vi "uTTA_Calibration_DiffAmp.vi"(6 "AR488_in":refnum<visa-resource-name>, 7 "CommandQueue":refnum<queue>, 8 "error in":errorcluster, 9 "FunctionGen_In":refnum<visa-resource-name>, 10 "DataQueue":refnum<queue>, 11 "TDMS_FileIn":refnum<k34>) -> (0 "error out":errorcluster, 1 "FunctionGen_Out":refnum<visa-resource-name>, 2 "aborted":bool, 3 "TDMS_FileOut":refnum<k34>, 4 "AR488_out":refnum<visa-resource-name>)   [LabVIEW 2021]
uses:
  <vilib>/Utility/miscctls.llb/LVPointTypeDef.ctl
  <vilib>/Analysis/6fits.llb/Curve Fitting Criteria.ctl
  <vilib>/Analysis/NI_AALPro.lvlib
panel:
  in  "START":bool
  out "ADC_Values":dbl[](array[numeric]) format="%#.2g"
  out "ADC_Variance":dbl[](array[numeric]) format="%#.2g"
  out "ADC offset":dbl format="%#_6pV"
  out "ADC lin. res":dbl caption="Residue" format="%.3p"
  out "ADC slope":dbl format="%#_4pV/Digit"
  out "Ref. Voltage":dbl format="%#_6pV"
  out "ADC Cal.":cluster{"mean":dbl, "mean":dbl}(graph)
  out "PGA setting":u32
  out "Calibration of Channel":u32
  in  "DAC Increments":dbl=0.05 caption="DAC Voltage Increment" min=0.001 max=1.0 format="%.3p V/Step"
  in  "Cal Adapter":bool=TRUE
  out "Status":string="Exit"
  in  "abort":bool
  # "1. Connect the function generator with a 50Ohm Terminator and a BNC Y-Adaptor to the input of the uTTA.\n2. Connect a ground lead to the outer Conductor of the BNC line to provide propper grounding\n3. Start the calibration"
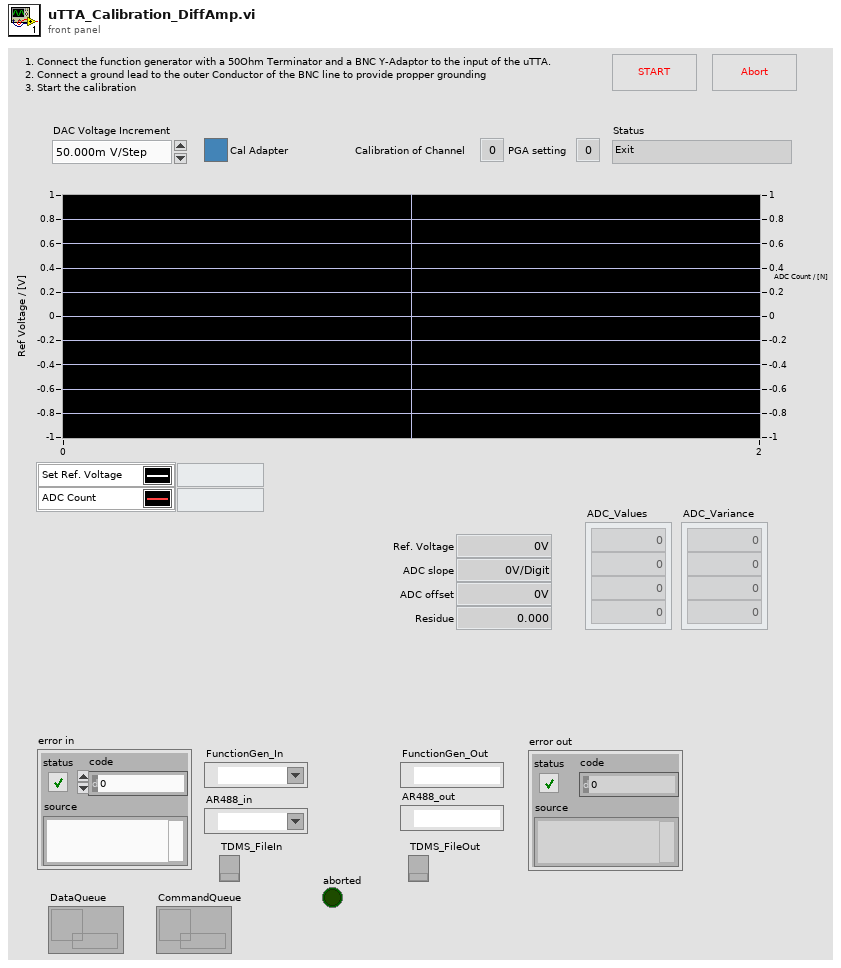
[diagram p1: front panel]
types:
  T1 = typedef "LVPointTypeDef.ctl" = cluster{"Horizontal":i16, "Vertical":i16}
  T2 = typedef "NI_AALPro.lvlib/Curve Fitting Criteria.ctl" = u16
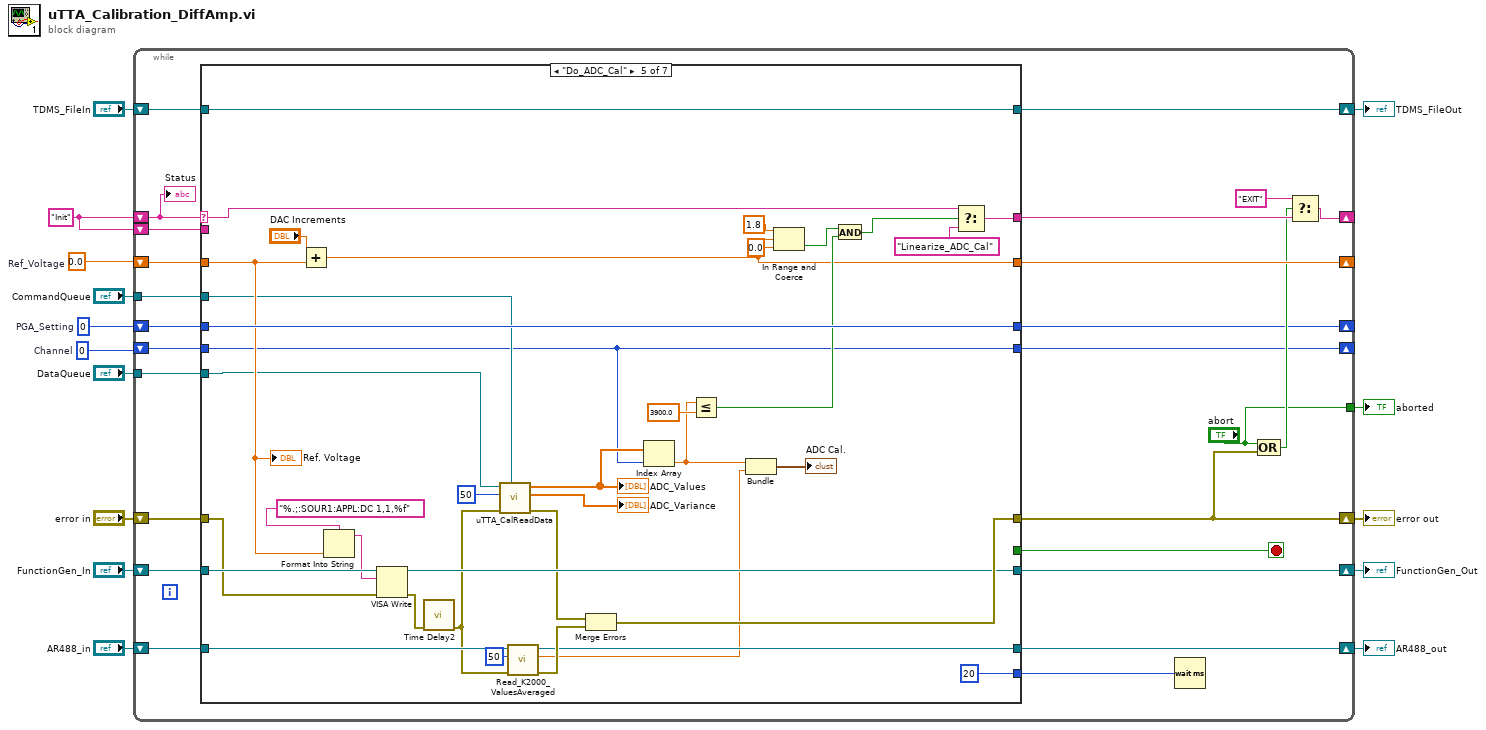
[diagram p0: block diagram]
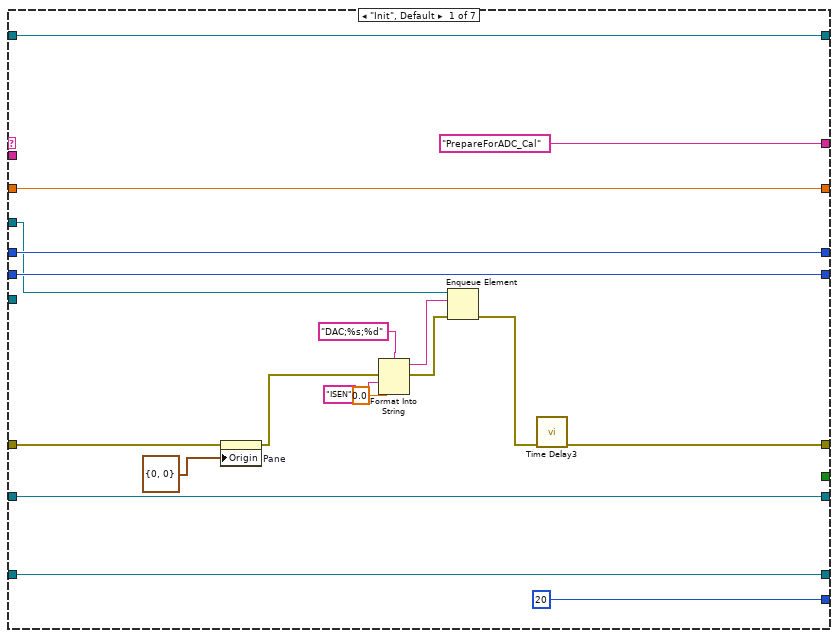
[diagram p2: hidden frame]
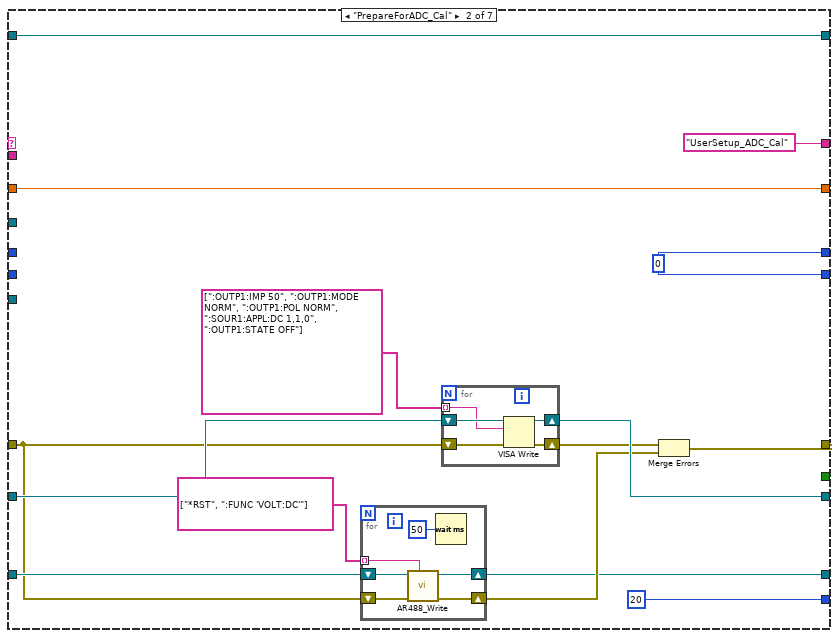
[diagram p3: hidden frame]
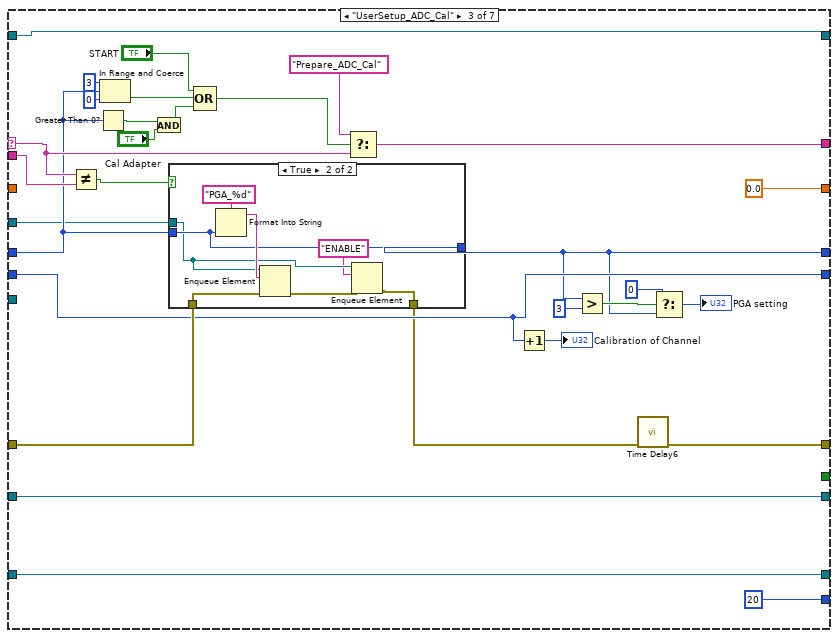
[diagram p4: hidden frame]
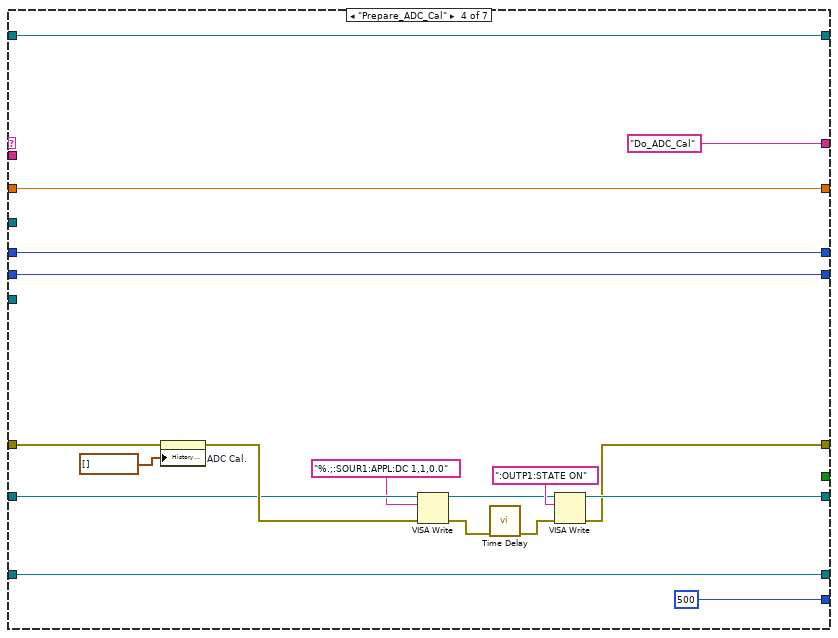
[diagram p6: hidden frame]
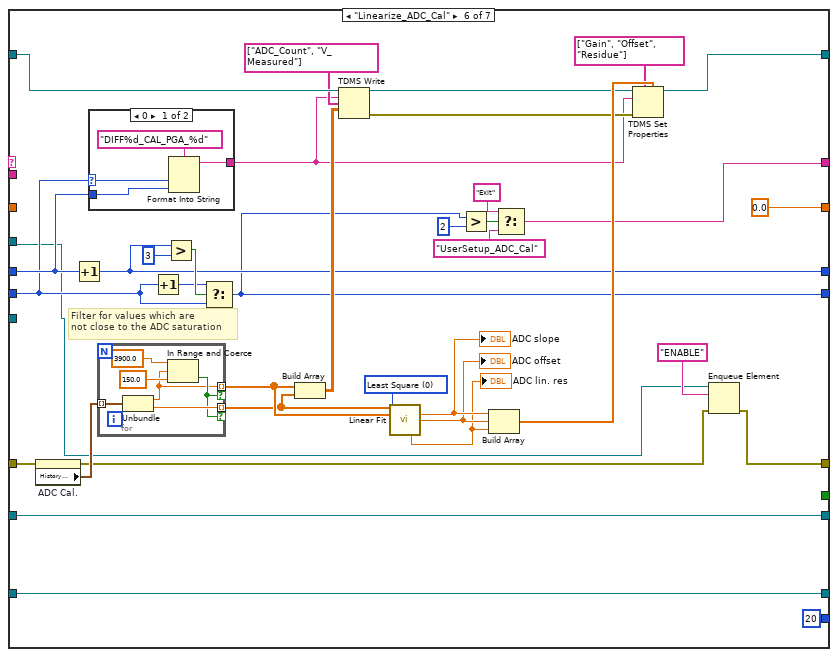
[diagram p7: hidden frame]
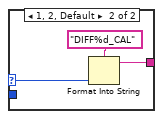
[diagram p8: hidden frame]
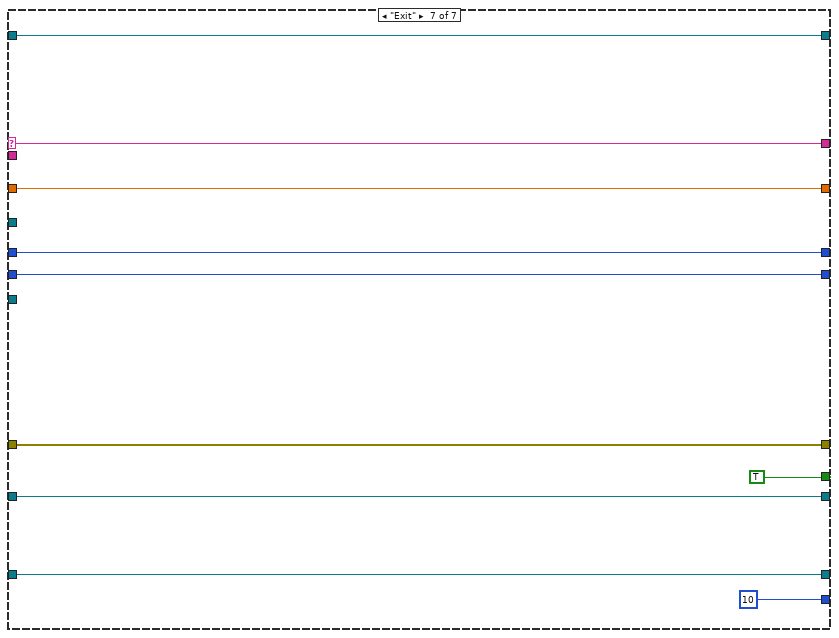
[diagram p9: hidden frame]
diagram:
  w11 = 0  # Channel
  w12 = 0  # PGA_Setting
  w14 = 0.0  # Ref_Voltage
  w13 = "Init"
  n1 = while {
    shift-right: [w27] -> _
    shift-left: w13 -> [w38]
    shift-right: [w25] -> w15
    shift-left: "error in" -> [w40]
    shift-right: [w36] -> w3
    shift-left: "FunctionGen_In" -> [w37]
    shift-right: [w35] -> w2
    shift-left: "AR488_in" -> [w34]
    shift-left: w13 -> [w33]
    tunnel: "CommandQueue" -> [w32]
    tunnel: "DataQueue" -> [w31]
    shift-right: [w29] -> _
    shift-left: w14 -> [w30]
    shift-right: [w22] -> w7
    shift-left: "TDMS_FileIn" -> [w21]
    shift-right: [w19] -> _
    shift-left: w12 -> [w20]
    shift-right: [w17] -> _
    shift-left: w11 -> [w18]
    tunnel: ["abort"] -> w1
    stop <- w23 stop-if-true
    n2 = case shown="\"Do_ADC_Cal\"" w38 {
      selector: w38 -> [_ _ w100 _ w175 _ w240]
      tunnel: [_ _ _ _ _ _ TRUE] -> w23
      tunnel: w40 -> [w56 w62 w108 w139 w165 w211 w234]
      tunnel: ["PrepareForADC_Cal" ("t") "UserSetup_ADC_Cal" ("t") w115 "Do_ADC_Cal" ("t") w174 w187 w240] -> w28
      tunnel: [w41 w71 w96 w135 w173 w183 w234] -> w25
      tunnel: [u32 20 u32 20 u32 20 u32 500 u32 20 u32 20 u32 10] -> w39
      tunnel: w37 -> [w55 w63 w114 w130 w166 w215 w233]
      tunnel: [w55 w73 w114 w136 w164 w215 w233] -> w36
      tunnel: [w54 w66 w113 w142 w169 w213 w232] -> w35
      tunnel: w34 -> [w54 w65 w113 w142 w171 w213 w232]
      tunnel: w33 -> [_ _ w99 _ _ _ _]
      tunnel: w32 -> [w43 _ w87 _ w145 w181 _]
      tunnel: w31 -> [_ _ _ _ w152 _ _]
      tunnel: w30 -> [w53 w70 _ w140 w154 _ w237]
      tunnel: [w53 w70 0.0 w140 w153 0.0 w237] -> w29
      tunnel: [w52 w64 w109 w138 w167 w209 w236] -> w22
      tunnel: w21 -> [w52 w64 w109 w138 w167 w210 w236]
      tunnel: w20 -> [w50 _ w94 w134 w159 w192 w231]
      tunnel: [w50 w60 w97 w134 w159 w199 w231] -> w19
      tunnel: w18 -> [w51 _ w104 w132 w144 w190 w235]
      tunnel: [w51 w60 w104 w132 w144 w188 w235] -> w17
      frame "Init", Default {
        n3 = property on="Pane" class="Pane"(error in=w56, "Origin"=T1 {"Horizontal"=0, "Vertical"=0}) -> (error out=w45:errorcluster)  [unwired: 1 in, 1 out]
        n4 = Format Into String(format string="DAC;%s;%d" ("element"), error in=w45, "ISEN" ("input 1"), 0.0 ("input 2")) -> (resulting string=w49:string, error out=w48:errorcluster)  [unwired: 1 in]
        n5 = Enqueue Element(queue=w43, element=w49, error in (no error)=w48) -> (error out=w42:errorcluster)  [unwired: 1 in, 2 out]
        n6 = call "Time Delay3"("error in (no error)"=w42) -> ("error out"=w41:errorcluster)  [unwired: 10 in]
      }
      frame "PrepareForADC_Cal" {
        w60 = 0 ("Channel")
        n7 = for {
          tunnel: string[] ["*RST", ":FUNC 'VOLT:DC'"] -> [w79] mode=indexing
          shift-right: [w77] -> w66
          shift-left: w65 -> [w80]
          shift-right: [w76] -> w67
          shift-left: w62 -> [w78]
          n8 = call "AR488_Write.vi"("write"=w79, "error in (no error)"=w78, "VISA Refnum in"=w80) -> ("error out"=w76:errorcluster, "VISA Refnum out"=w77:refnum<visa-resource-name>)  [unwired: 7 in]
          n9 = Wait (ms)(milliseconds to wait=u32 50) -> ()  [unwired: 1 out]
        }
        n10 = for {
          shift-right: [w84] -> w73
          shift-left: w63 -> [w85]
          tunnel: string[] [":OUTP1:IMP 50", ":OUTP1:MODE NORM", ":OUTP1:POL NORM", ":SOUR1:APPL:DC 1,1,0", ":OUTP1:STATE OFF"] ("Array 2") -> [w83] mode=indexing
          shift-right: [w81] -> w72
          shift-left: w62 -> [w82]
          n11 = VISA Write(VISA resource name=w85, write buffer=w83, error in (no error)=w82) -> (VISA resource name out=w84:refnum<visa-resource-name>, error out=w81:errorcluster)  [unwired: 1 out]
        }
        n12 = Merge Errors(w72, w67) -> (w71:errorcluster)
      }
      frame "UserSetup_ADC_Cal" {
        n13 = Not Equal?(x=w100, y=w99) -> (x != y?=w98:bool)
        n14 = Greater Than 0?(x=w94) -> (x > 0?=w92:bool)
        n15 = In Range and Coerce(upper limit=u32 3, x=w94, lower limit=u32 0) -> (In Range?=w101:bool)  [unwired: 1 out]
        n16 = And(x=w92, y="Cal Adapter") -> (x .and. y?=w91:bool)
        n17 = case shown="True" w98 {
          tunnel: w108 -> [w116 w125]
          tunnel: w87 -> [_ w121]
          tunnel: w94 -> [w117 w122]
          tunnel: [w117 w122] -> w97
          tunnel: [w116 w118] -> w86
          frame False {
          }
          frame True {
            n18 = Format Into String(format string="PGA_%d" ("element"), w122) -> (resulting string=w123:string)  [unwired: 2 in, 1 out]
            n19 = Enqueue Element(queue=w121, element=w123, error in (no error)=w125) -> (error out=w119:errorcluster)  [unwired: 1 in, 2 out]
            n20 = Enqueue Element(queue=w121, element="ENABLE", error in (no error)=w119) -> (error out=w118:errorcluster)  [unwired: 1 in, 2 out]
          }
        }
        n21 = Compound Arithmetic op=OR("START", w101, w91) -> (w103:bool)
        n22 = Select(t="Prepare_ADC_Cal", s=w103, f=w100) -> (s? t:f=w115:string)
        n23 = Increment(x=w104) -> (x+1=→"Calibration of Channel":i32)
        n24 = Greater?(x=w97, y=u32 3) -> (0:w106:bool)
        n25 = call "Time Delay6"("error in (no error)"=w86) -> ("error out"=w96:errorcluster)  [unwired: 10 in]
        n26 = Select(t=u32 0, s=w106, f=w97) -> (s? t:f=→"PGA setting":u32)
      }
      frame "Prepare_ADC_Cal" {
        n27 = property on="ADC Cal." class="WFChart (strict)"(error in=w139, "History Data"=cluster{"Voltage mean":dbl, "mean":dbl}[] []) -> (error out=w131:errorcluster)  [unwired: 1 in, 1 out]
        n28 = VISA Write(VISA resource name=w130, write buffer="%.;:SOUR1:APPL:DC 1,1,0.0", error in (no error)=w131) -> (VISA resource name out=w128:refnum<visa-resource-name>, error out=w127:errorcluster)  [unwired: 1 out]
        n29 = call "Time Delay"("error in (no error)"=w127) -> ("error out"=w126:errorcluster)  [unwired: 10 in]
        n30 = VISA Write(VISA resource name=w128, write buffer=":OUTP1:STATE ON", error in (no error)=w126) -> (VISA resource name out=w136:refnum<visa-resource-name>, error out=w135:errorcluster)  [unwired: 1 out]
      }
      frame "Do_ADC_Cal" {
        n31 = Add(x="DAC Increments", y=w154) -> (x+y=w153:dbl)
        n32 = Format Into String(format string="%.;:SOUR1:APPL:DC 1,1,%f" ("write buffer"), w154) -> (resulting string=w161:string)  [unwired: 2 in, 1 out]
        n33 = VISA Write(VISA resource name=w166, write buffer=w161, error in (no error)=w165) -> (VISA resource name out=w164:refnum<visa-resource-name>, error out=w163:errorcluster)  [unwired: 1 out]
        n34 = call "Time Delay2"("error in (no error)"=w163) -> ("error out"=w151:errorcluster)  [unwired: 10 in]
        n35 = call "uTTA_CalReadData.vi"("Control Queue"=w145, "error in"=w151, "Averaged Values"=50, "Data Queue in"=w152) -> ("error out"=w150:errorcluster, "ADC_Variance"=→"ADC_Variance":dbl[], "ADC_Values"=w147:dbl[])  [unwired: 3 in, 2 out]
        "ADC_Values" <- w147
        n36 = call "Read_K2000_ValuesAveraged.vi"("error in"=w151, "No. Averaged Values"=50, "VISA Refnum in"=w171) -> ("error out"=w170:errorcluster, "mean"=w160:dbl, "VISA Refnum out"=w169:refnum<visa-resource-name>)  [unwired: 6 in]
        n37 = Merge Errors(w150, w170) -> (w173:errorcluster)
        n38 = Index Array(array=w147, index=w144) -> (element=w146:dbl)
        n39 = Less Or Equal?(x=w146, y=3900.0) -> (x <= y?=w157:bool)
        n40 = Bundle("mean"=w146, "mean"=w160) -> (→"ADC Cal.":cluster{"mean":dbl, "mean":dbl})  [unwired: 1 in]
        n41 = In Range and Coerce(upper limit=1.8, x=w153, lower limit=0.0) -> (In Range?=w156:bool)  [unwired: 1 out]
        n42 = And(x=w156, y=w157) -> (x .and. y?=w155:bool)
        n43 = Select(t=w175, s=w155, f="Linearize_ADC_Cal") -> (s? t:f=w174:string)
        "Ref. Voltage" <- w154
      }
      frame "Linearize_ADC_Cal" {
        w216 = T2 0 items=["Least Square", "Least Absolute Residual", "Bisquare"] ("method")
        # "Filter for values which are \nnot close to the ADC saturation"
        n44 = property on="ADC Cal." class="WFChart (strict)"(error in=w211) -> (error out=w184:errorcluster, "History Data"=w217:cluster{"Voltage mean":dbl, "mean":dbl}[])  [unwired: 1 in, 1 out]
        n45 = Increment(x=w192) -> (x+1=w199:i32)
        n46 = case shown="0" w190 {
          selector: w190 -> [w219 w222]
          tunnel: w192 -> [w218 _]
          tunnel: [w220 w223] -> w191
          frame 0 {
            n47 = Format Into String(format string="DIFF%d_CAL_PGA_%d" ("group name in (Untitled)"), w219, w218) -> (resulting string=w220:string)  [unwired: 2 in, 1 out]
          }
          frame 1, 2, Default {
            n48 = Format Into String(format string="DIFF%d_CAL" ("group name in (Untitled)"), w222) -> (resulting string=w223:string)  [unwired: 2 in, 1 out]
          }
        }
        n49 = for {
          tunnel: w217 -> [w230] mode=indexing
          tunnel: [w229] -> w185 mode=indexing if=w227
          tunnel: [w226] -> w186 mode=indexing if=w227
          n50 = Unbundle(w230) -> ("Voltage mean"=w226:dbl, "mean"=w229:dbl)
          n51 = In Range and Coerce(upper limit=3900.0, x=w226, lower limit=150.0 ("y")) -> (In Range?=w227:bool)  [unwired: 1 out]
        }
        n52 = Increment(x=w190) -> (x+1=w200:i32)
        n53 = Greater?(x=w199, y=u32 3) -> (0:w201:bool)
        n54 = Select(t=w200, s=w201, f=w190) -> (s? t:f=w188:i32)
        n55 = Build Array(w186, w185) -> (w208:dbl[][])
        n56 = TDMS Write(0:w210, 5:w191, 7:string[] ["ADC_Count", "V_Measured"], 9:w208) -> (4:w195:refnum<k34>, 15:w194:errorcluster)  [unwired: 2 in, 2 out]
        n57 = call <vilib>:"Linear Fit.vi"("Y"=w185, "X"=w186, "method"=w216) -> ("slope"=w207:dbl, "intercept"=w206:dbl, "residue"=w189:dbl)  [unwired: 8 in, 2 out]
        "ADC offset" <- w206
        "ADC lin. res" <- w189
        "ADC slope" <- w207
        n58 = Greater?(x=w188, y=u32 2) -> (0:w197:bool)
        n59 = Build Array(w207, w206, w189) -> (w205:dbl[])
        n60 = Select(t="Exit", s=w197, f="UserSetup_ADC_Cal" ("t")) -> (s? t:f=w187:string)
        n61 = TDMS Set Properties(5:w205, 7:string[] ["Gain", "Offset", "Residue"] ("property names"), 8:w194, 10:w191, 11:w195) -> (3:w209:refnum<k34>)  [unwired: 1 in, 3 out]
        n62 = Enqueue Element(queue=w181, element="ENABLE", error in (no error)=w184) -> (error out=w183:errorcluster)  [unwired: 1 in, 2 out]
      }
      frame "Exit" {
      }
    }
    n63 = Wait (ms)(milliseconds to wait=w39) -> ()  [unwired: 1 out]
    n64 = Compound Arithmetic op=OR("abort", w25) -> (w24:bool)
    n65 = Select(t="EXIT", s=w24, f=w28) -> (s? t:f=w27:string)
    "Status" <- w38
  }
  "TDMS_FileOut" <- w7
  "error out" <- w15
  "FunctionGen_Out" <- w3
  "AR488_out" <- w2
  "aborted" <- w1
